vi "Text to UTF-8 (LabVIEW Path).vi"(8 "error in":errorcluster, 10 "Encoding (system default=-1)":i32=-1, 11 "Path":path) -> (0 "error out":errorcluster, 3 "UTF-8 Encoded Path":T1)   [LabVIEW 2020, in "G-Unicode.lvlib"]
uses:
  G-Unicode.lvlib
  Types/Encoded UTF-8 Path.ctl
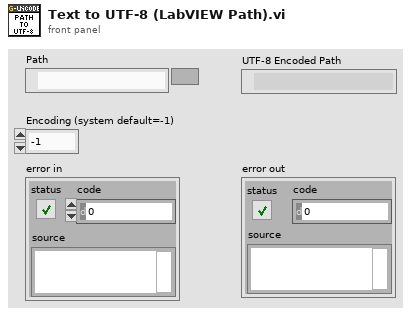
[diagram p1: front panel]
types:
  T1 = typedef "G-Unicode.lvlib/Encoded UTF-8 Path.ctl" = path
  T2 = typedef "G-Unicode.lvlib/Encoded UTF-8 String.ctl" = string
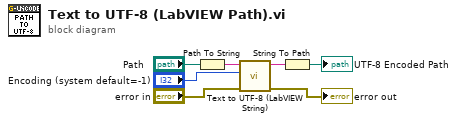
[diagram p0: block diagram]
diagram:
  n1 = Path To String(path="Path") -> (string=w2:string)
  n2 = call "Text to UTF-8 (LabVIEW String).vi"("error in"="error in", "Encoding (system default=-1)"="Encoding (system default=-1)", "String"=w2) -> ("error out"=→"error out":errorcluster, "UTF-8 Encoded String"=w3:T2)  [unwired: 7 in]
  n3 = String To Path(string=w3) -> (path=→"UTF-8 Encoded Path":path)
